vi "GetCtrlName.vi"(2 "Control Data":variant) -> (4 "found":bool, 6 "Ctrl Label":string, 7 "Data":variant)   [LabVIEW 2025, in "UI_Library.lvlib" / "UI_Library.lvclass"]
doc: "Get Control Label"
uses:
  UI_Library.lvclass
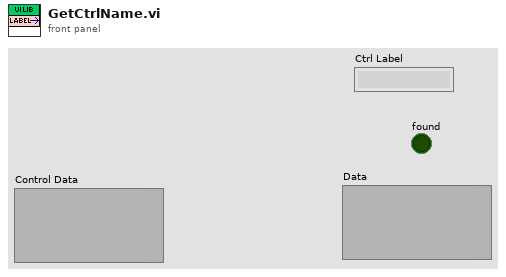
[diagram p1: front panel]
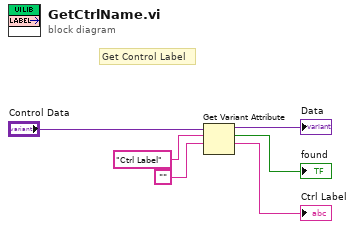
[diagram p0: block diagram]
diagram:
  # "Get Control Label"
  n1 = Get Variant Attribute(Variant="Control Data", name="Ctrl Label" ("Control Label"), default value (empty Variant)="") -> (duplicate Variant=→"Data":variant, found=→"found":bool, value=→"Ctrl Label":string)  [unwired: 1 in, 1 out]
